vi "mult_process.vi"() -> ()   [LabVIEW 2013]
uses:
  results_cluster.ctl
  <vilib>/Utility/file.llb/Read From Spreadsheet File (DBL).vi
  <vilib>/gmath/statdist.llb/Student t Inverse CDF.vi
  <vilib>/Analysis/NI_AALBase.lvlib
  <vilib>/gmath/NI_Gmath.lvlib
panel:
  in  "Значимость":dbl
  in  "Путь":path caption="Путь к файлу"
  in  "Строка форматирования":string="%_5f ± %_3f; %_2f"
  out "Результат измерений":string
  in  "Pдов":dbl=0.95
  in  "Границы НСП":dbl
  out "Результаты обработки":T1 {"Dдов рез" format="%#.4g"; "S сумм" format="%#.4g"; "К" format="%#.4g"; "Dдов случ." format="%#.4g"; "Sхср" format="%#.4g"; "S" format="%#.4g"}
  in  "Записать результат":bool
  in  "Получить данные":bool
  in  "Вычислить Dдов":bool
  out "Ряд измерений":dbl[](graph)
  in  "Стоп":bool
  in  "Вычислить оценки":bool
  # "Обработка результатов многократных измерений"
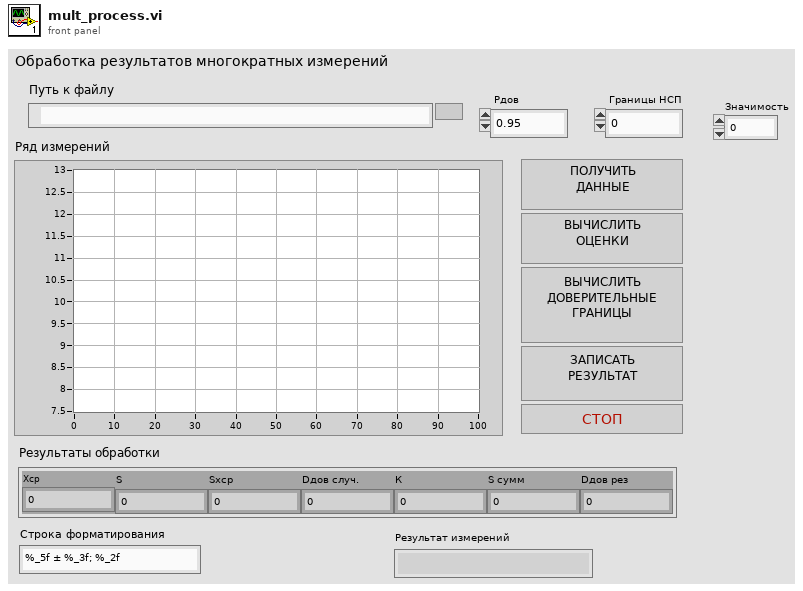
[diagram p1: front panel]
types:
  T1 = typedef "results_cluster.ctl" = cluster{"Xср":dbl, "S":dbl, "Sхср":dbl, "Dдов случ.":dbl, "К":dbl, "S сумм":dbl, "Dдов рез":dbl}
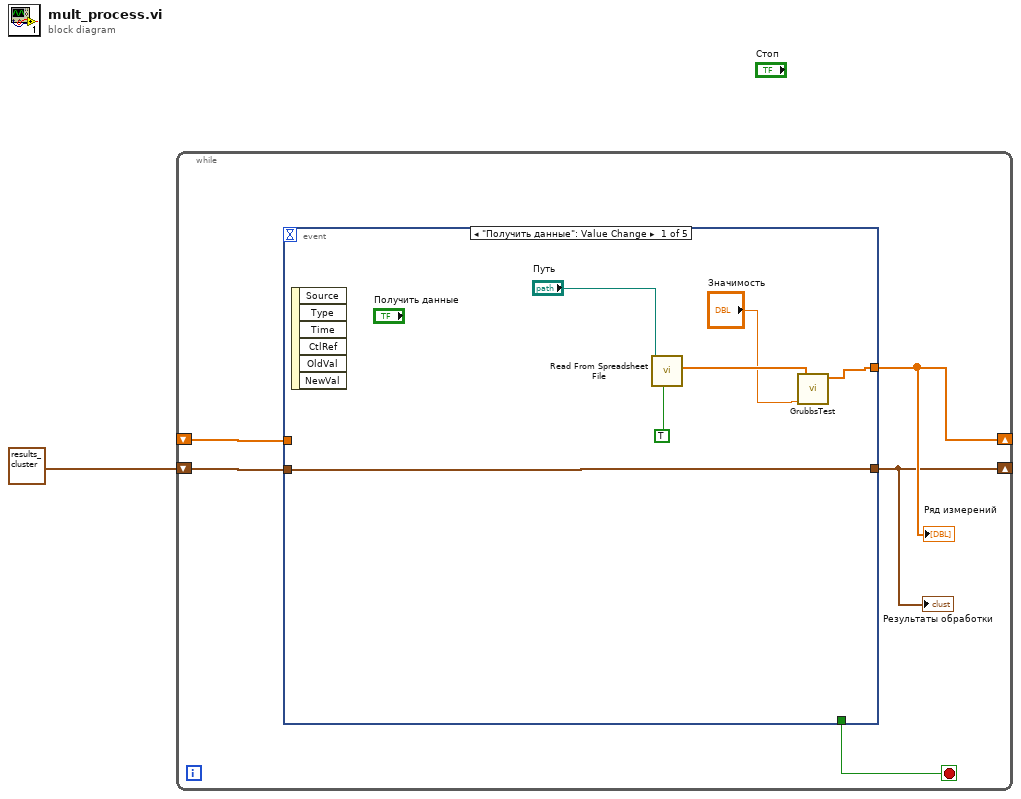
[diagram p0: block diagram]
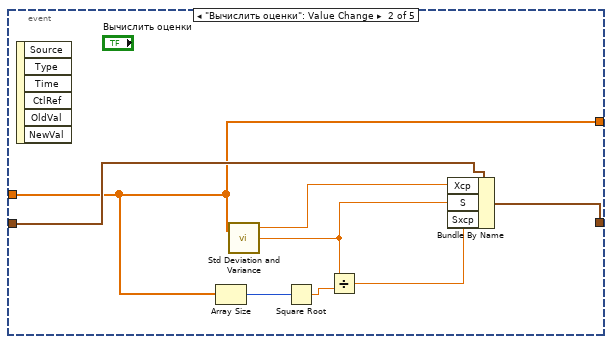
[diagram p2: hidden frame]
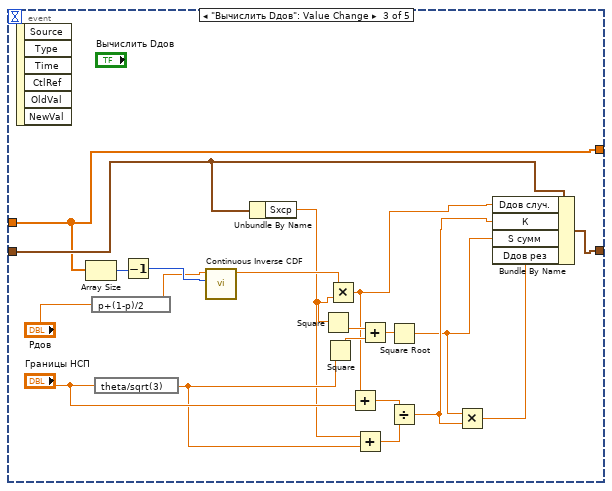
[diagram p3: hidden frame]
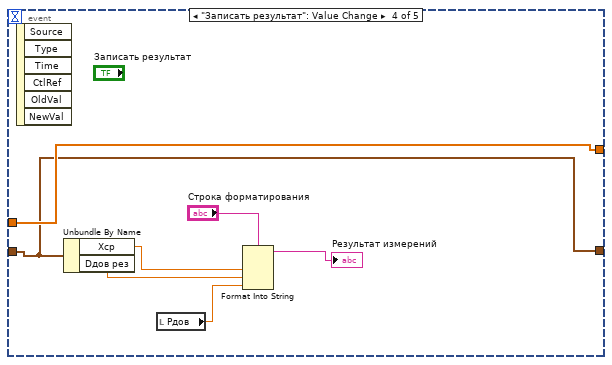
[diagram p4: hidden frame]
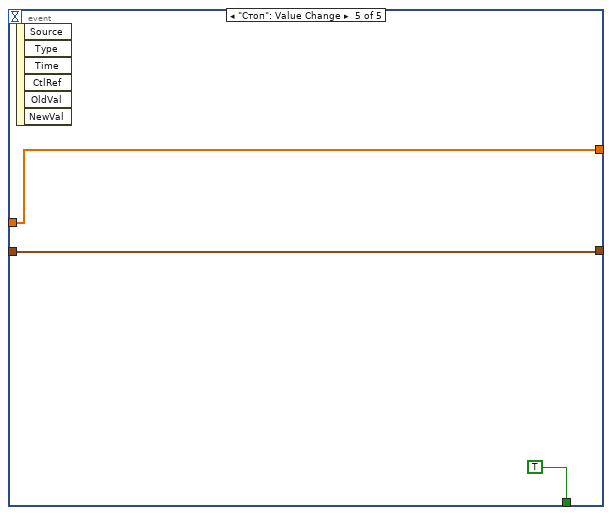
[diagram p5: hidden frame]
diagram:
  n1 = while {
    shift-right: [w3] -> _
    shift-left: _ -> [w6]
    shift-right: [w2] -> _
    shift-left: T1 {"Xср"=1.3199999999999998, "S"=0.130384048104053, "Sхср"=0.05830951894845301, "Dдов случ."=0.16189317847087023, "К"=2.43060784036949, "S сумм"=0.06506407098647712, "Dдов рез"=0.15814524106608838} ("Результаты обработки") -> [w5]
    stop <- w4 stop-if-true
    n2 = event shown="[0] \"Получить данные\": Value Change" {
      selector: _ -> [_ _ _ _ _]
      dyn-events: _ -> [_ _ _ _ _]
      timeout: _ -> [_ _ _ _ _]
      tunnel: w6 -> [_ w13 w39 w47 w50]
      tunnel: w5 -> [w10 w16 w40 w41 w49]
      tunnel: [w10 w15 w21 w41 w49] -> w2
      tunnel: [w7 w13 w39 w47 w50] -> w3
      tunnel: [_ _ _ _ TRUE] -> w4
      event "Получить данные": Value Change {
        n3 = event-data() -> ()  [unwired: 1 in, 6 out]
        n4 = call-poly <vilib>:"Read From Spreadsheet File.vi"("transpose (no:F)"=TRUE, "file path (dialog if empty)"="Путь") -> ("first row"=w9:dbl[])  [unwired: 5 in, 4 out]
        n5 = call "GrubbsTest.vi"("Значимость"="Значимость", "Исходные"=w9) -> ("Обработанные"=w7:dbl[])  [unwired: 2 in, 3 out]
      }
      event "Вычислить оценки": Value Change {
        n6 = event-data() -> ()  [unwired: 1 in, 6 out]
        n7 = Array Size(array=w13) -> (size(s)=w14:i32)
        n8 = call <vilib>:"Std Deviation and Variance.vi"("X"=w13) -> ("mean"=w17:dbl, "standard deviation"=w18:dbl)  [unwired: 1 in, 1 out]
        n9 = Square Root(x=w14) -> (sqrt(x)=w20:dbl)
        n10 = Divide(x=w18, y=w20) -> (x/y=w19:dbl)
        n11 = Bundle By Name(cluster=w16, "Xср"=w17, "S"=w18, "Sхср"=w19) -> (w15:T1)
      }
      event "Вычислить Dдов": Value Change {
        n12 = event-data() -> ()  [unwired: 1 in, 6 out]
        n13 = Array Size(array=w39) -> (size(s)=w38:i32)
        n14 = expression code="p+(1-p)/2"("Pдов") -> (w36:dbl)
        n15 = expression code="theta/sqrt(3)"("Границы НСП") -> (w28:dbl)
        n16 = Decrement(x=w38) -> (x-1=w37:i32)
        n17 = call-poly <vilib>:"Continuous Inverse CDF.vi"("k degrees of freedom"=w37, "cdf(x)"=w36) -> ("x"=w34:dbl)  [unwired: 8 in, 1 out]
        n18 = Unbundle By Name(w40) -> ("Sхср"=w27:dbl)
        n19 = Square(x=w27) -> (x^2=w32:dbl)
        n20 = Square(x=w28) -> (x^2=w33:dbl)
        n21 = Multiply(x=w34, y=w27) -> (x*y=w29:dbl)
        n22 = Add(x=w29, y="Границы НСП") -> (x+y=w26:dbl)
        n23 = Add(x=w27, y=w28) -> (x+y=w25:dbl)
        n24 = Add(x=w32, y=w33) -> (x+y=w31:dbl)
        n25 = Square Root(x=w31) -> (sqrt(x)=w23:dbl)
        n26 = Divide(x=w26, y=w25) -> (x/y=w24:dbl)
        n27 = Multiply(x=w23, y=w24) -> (x*y=w22:dbl)
        n28 = Bundle By Name(cluster=w40, "Dдов случ."=w29, "К"=w24, "S сумм"=w23, "Dдов рез"=w22) -> (w21:T1)
      }
      event "Записать результат": Value Change {
        n29 = event-data() -> ()  [unwired: 1 in, 6 out]
        n30 = Unbundle By Name(w41) -> ("Xср"=w43:dbl, "Dдов рез"=w42:dbl)
        n31 = local read "Pдов"() -> (w45:dbl)
        n32 = Format Into String(format string="Строка форматирования", w43, w42, w45) -> (resulting string=→"Результат измерений":string)  [unwired: 2 in, 1 out]
      }
      event "Стоп": Value Change {
        n33 = event-data() -> ()  [unwired: 1 in, 6 out]
      }
    }
    "Ряд измерений" <- w3
    "Результаты обработки" <- w2
  }
